vi "nth Derivative of Polynomial (DBL).vi"(10 "order":i32, 11 "P(x)":dbl[](array[numeric]) min=0.0 max=127.0 format="%#.6g") -> (0 "error":i32, 3 "Nth Derivative of P(x)":dbl[](array[numeric]) min=0.0 max=127.0 format="%#.6g")   [LabVIEW 2020, in "NI_AALPro.lvlib"]
doc: "Calculates the nth order derivative of <B>P(x)</B>. Wire data to the <B>P(x)</B> input to determine the polymorphic instance to use or manually select the instance."
uses:
  <vilib>/Analysis/NI_AALPro.lvlib
  <vilib>/Analysis/polynomials.llb/Remove Zero Coefficients (DBL).vi
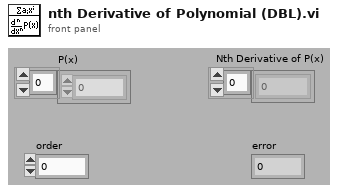
[diagram p1: front panel]
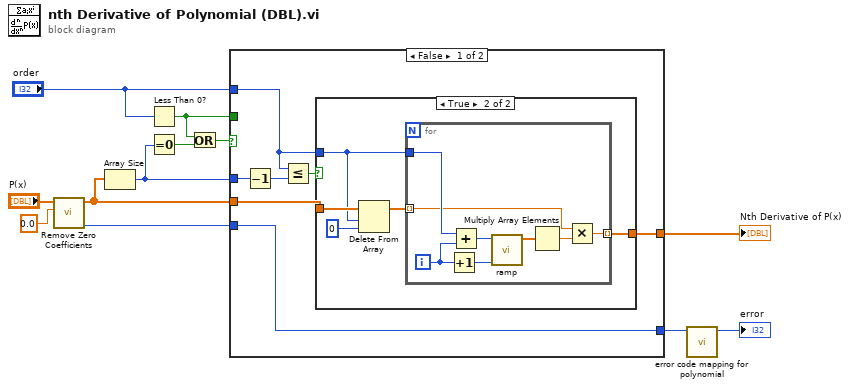
[diagram p0: block diagram]
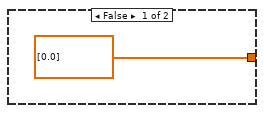
[diagram p2: hidden frame]
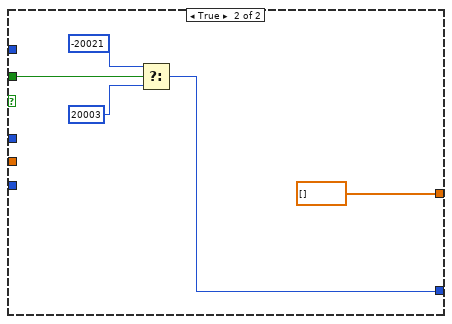
[diagram p3: hidden frame]
diagram:
  n1 = call-poly <vilib>:"Remove Zero Coefficients.vi"("threshold"=0.0, "P(x) In"="P(x)") -> ("error"=w3:i32, "P(x) Out"=w11:dbl[])  [unwired: 7 in, 1 out]
  n2 = Array Size(array=w11) -> (size(s)=w10:i32)
  n3 = Less Than 0?(x="order") -> (x < 0?=w5:bool)
  n4 = Equal To 0?(x=w10) -> (x = 0?=w8:bool)
  n5 = Or(x=w5, y=w8) -> (x .or. y?=w7:bool)
  n6 = case shown="False" w7 {
    tunnel: w11 -> [w19 _]
    tunnel: w10 -> [w16 _]
    tunnel: "order" -> [w15 _]
    tunnel: [w13 w36] -> w2
    tunnel: [w14 dbl[] []] -> w6
    tunnel: w5 -> [_ w37]
    tunnel: w3 -> [w13 _]
    frame False {
      n7 = Decrement(x=w16) -> (x-1=w17:i32)
      n8 = Less Or Equal?(x=w15, y=w17) -> (x <= y?=w18:bool)
      n9 = case shown="True" w18 {
        tunnel: w19 -> [_ w25]
        tunnel: w15 -> [_ w23]
        tunnel: [dbl[] [0.0] ("Polynomial dp(s)/ds") w21] -> w14
        frame False {
        }
        frame True {
          n10 = Delete From Array(array=w25, length=w23, index=0) -> (array with subset deleted=w22:dbl[])  [unwired: 1 out]
          n11 = for {
            tunnel: w22 -> [w31] mode=indexing
            tunnel: w23 -> [w32]
            tunnel: [w29] -> w21 mode=indexing
            i -> [w33]
            n12 = Increment(x=w33) -> (x+1=w27:i32)
            n13 = Add(x=w32, y=w33) -> (x+y=w28:i32)
            n14 = call <vilib>:"ramp.vi"("start"=w27, "end"=w28) -> ("ramp"=w26:dbl[])  [unwired: 9 in]
            n15 = Multiply Array Elements(1:w26) -> (0:w30:dbl)
            n16 = Multiply(x=w31, y=w30) -> (x*y=w29:dbl)
          }
        }
      }
    }
    frame True {
      n17 = Select(t=-20021 ("minus order"), s=w37, f=20003 ("empty array")) -> (s? t:f=w36:i32)
    }
  }
  "Nth Derivative of P(x)" <- w6
  n18 = call <vilib>:"error code mapping for polynomial.vi"("error in"=w2) -> ("error out"=→"error":i32)  [unwired: 10 in]
